vi "Error2XML.vi"(1 "FailDescriptor":string, 2 "FailID":i32) -> (0 "ErrorXML":string)   [LabVIEW 2010]
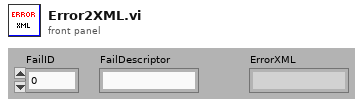
[diagram p1: front panel]
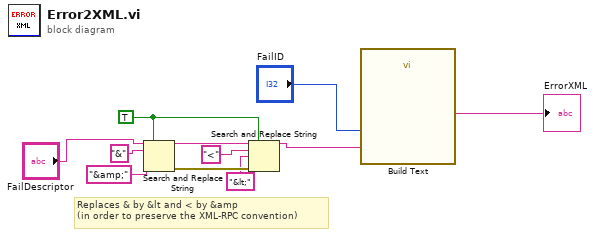
[diagram p0: block diagram]
diagram:
  w1 = TRUE ("replace all? (F)")
  # "Replaces & by &lt and < by &amp\n(in order to preserve the XML-RPC convention)"
  n1 = Search and Replace String(replace all?=w1, input string="FailDescriptor", search string="&", replace string="&amp;" ("replace string (\"\")")) -> (result string=w9:string, error out=w8:errorcluster)  [unwired: 4 in, 2 out]
  n2 = Search and Replace String(replace all?=w1, input string=w9, search string="<", replace string="&lt;" ("replace string (\"\")"), error in=w8) -> (result string=w3:string)  [unwired: 3 in, 3 out]
  n3 = call "Build Text"("FailID"="FailID", "FailDescriptor"=w3) -> ("Result"=→"ErrorXML":string)  [unwired: 12 in, 1 out]
